vi "daq-BackUp.vi"() -> ()   [LabVIEW 2014]
uses:
  <vilib>/DAQmx/write.llb/DAQmx Write (Digital 1D Bool NChan 1Samp 1Line).vi
  <vilib>/DAQmx/read.llb/DAQmx Read (Digital 1D Bool NChan 1Samp 1Line).vi
panel:
  in  "Ignore Memory?":bool
  in  "Reset":bool
  in  "LED --> Motor":bool
  in  "Backward":bool
  in  "Forward":bool
  out "LED?":bool
  in  "stop":bool
  # "Quiz 3:\nBuilding Electronic Circuits"
  # "P0.0 = Forward           (output)\nP0.1 = NOT Forward   (output)\nP0.2 = Backward         (output)\nP0.3 = NOT Backward (output)\nP0.4 = Reset               (output)\nP0.5 = LED                  ( input  )"
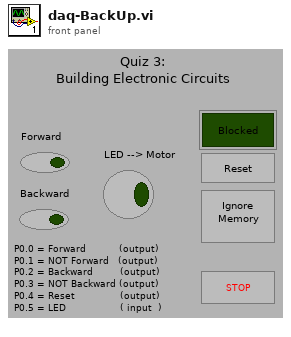
[diagram p1: front panel]
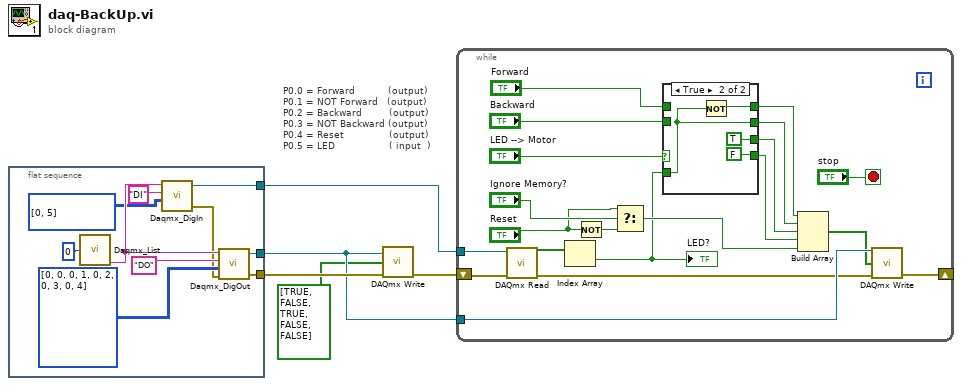
[diagram p0: block diagram]
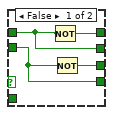
[diagram p2: hidden frame]
diagram:
  # "P0.0 = Forward           (output)\nP0.1 = NOT Forward   (output)\nP0.2 = Backward         (output)\nP0.3 = NOT Backward (output)\nP0.4 = Reset               (output)\nP0.5 = LED                  ( input  )"
  n1 = flat-sequence {
    tunnel: [w7] -> w5
    tunnel: [w11] -> w1
    tunnel: [w10] -> w3
    frame #0 {
      n2 = call "Daqmx_List.vi"("Device Number n"=u8 0) -> ("NI-DAQmx Device Name n"=w12:tag)  [unwired: 3 out]
      n3 = call "Daqmx_DigIn.vi"("Array of Ports, Lines"=i32[][] [[0, 5]] ("Outputs: Port, Line"), "Base Task Name"="DI", "DAQmx device name"=w12) -> ("error out"=w6:errorcluster, "Input Task Name"=w11:refnum<k21>)  [unwired: 1 in, 1 out]
      n4 = call "Daqmx_DigOut.vi"("error in"=w6, "Array of Ports, Lines"=i32[][] [[0, 0], [0, 1], [0, 2], [0, 3], [0, 4]] ("Inputs: Port, Line"), "Base Task Name"="DO", "DAQmx device name"=w12) -> ("error out"=w7:errorcluster, "Output Task Name"=w10:refnum<k21>)  [unwired: 1 out]
    }
  }
  n5 = call-poly <vilib>:"DAQmx Write.vi"("task/channels in"=w3, "data"=bool[] [TRUE, FALSE, TRUE, FALSE, FALSE], "error in"=w5) -> ("error out"=w4:errorcluster)  [unwired: 1 in, 11 out]
  n6 = while {
    tunnel: w1 -> [w34]
    tunnel: w3 -> [w32]
    shift-right: [w27] -> _
    shift-left: w4 -> [w29]
    stop <- "stop" stop-if-true
    n7 = call-poly <vilib>:"DAQmx Read.vi"("task/channels in"=w34, "error in"=w29) -> ("data"=w35:bool[], "error out"=w28:errorcluster)  [unwired: 1 in, 11 out]
    n8 = Index Array(array=w35) -> (element=w25:bool)  [unwired: 1 in]
    "LED?" <- w25
    n9 = Not(x="Reset") -> (.not. x?=w17:bool)
    n10 = Select(t="Reset", s="Ignore Memory?", f=w17) -> (s? t:f=w31:bool)
    n11 = case shown="True" "LED --> Motor" {
      tunnel: w25 -> [_ w42]
      tunnel: [w36 FALSE] -> w21
      tunnel: [w38 w42] -> w19
      tunnel: "Backward" -> [w36 _]
      tunnel: "Forward" -> [w38 _]
      tunnel: [w39 w43] -> w22
      tunnel: [w37 TRUE] -> w20
      frame False {
        n12 = Not(x=w38) -> (.not. x?=w39:bool)
        n13 = Not(x=w36) -> (.not. x?=w37:bool)
      }
      frame True {
        n14 = Not(x=w42) -> (.not. x?=w43:bool)
      }
    }
    n15 = Build Array(w22, w19, w20, w21, w31) -> (w30:bool[])
    n16 = call-poly <vilib>:"DAQmx Write.vi"("task/channels in"=w32, "data"=w30, "error in"=w28) -> ("error out"=w27:errorcluster)  [unwired: 1 in, 11 out]
  }
